vi "Query Multi Eval Meas Modulation Limit Check Results.vi"(8 "error in (no error)":errorcluster, 9 "Result Type (Current)":i32(ring) items=["Current", "Average", "Extreme"], 10 "Instance (1)":T1=1, 11 "VISA resource name":refnum<visa-resource-name>) -> (0 "error out":errorcluster, 1 "Modulation Limit Check Results":i32[](array[numeric]), 2 "Reliability":i32, 3 "VISA resource name out":refnum<visa-resource-name>)   [LabVIEW 2020, in "Rohde&Schwarz CMXP NR FR2 Measurement.lvlib"]
doc: "Starts a new single shot measurement and returns the multi eval measurement modulation results.\n\nAttributes:\nRSCMXPNRFR2M_ATTR_QUERY_MULTI_EVAL_MEASUREMENT_MODULATION_AVERAGE_LIMIT_CHECK_RESULTS\nRSCMXPNRFR2M_ATTR_QUERY_MULTI_EVAL_MEASUREMENT_MODULATION_CURRENT_LIMIT_CHECK_RESULTS\nRSCMXPNRFR2M_ATTR_QUERY_MULTI_EVAL_MEASUREMENT_MODULATION_EXTREME_LIMIT_CHECK_RESULTS\n\nRemote-control commands:\nCALCulate:NRMMw:MEAS<i>:MEValuation:MODulation:AVERage?\nCALCulate:NRMMw:MEAS<i>:MEValuation:MODulation:CURRent?\nCALCulate:NRMMw:MEAS<i>:MEValuation:MODulation:EXTReme?"
uses:
  <instrlib>/Rohde&Schwarz CMXP NR FR2 Measurement/Rohde&Schwarz CMXP NR FR2 Measurement.lvlib
  <instrlib>/Rohde&Schwarz CMXP NR FR2 Measurement/Private/_Instance.ctl
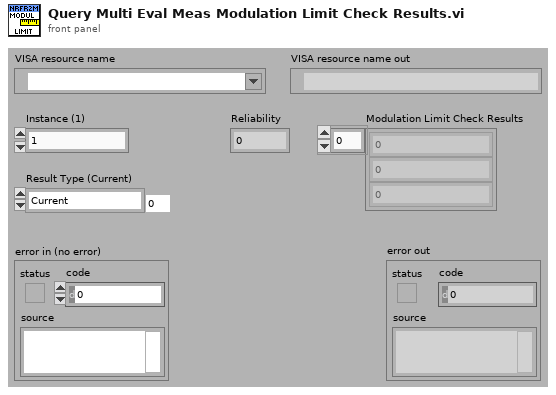
[diagram p1: front panel]
types:
  T1 = typedef "Rohde&Schwarz CMXP NR FR2 Measurement.lvlib/_Instance.ctl" = i32
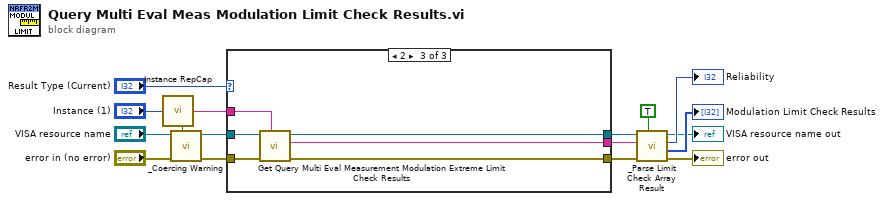
[diagram p0: block diagram]
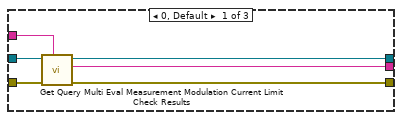
[diagram p2: hidden frame]
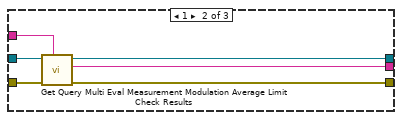
[diagram p3: hidden frame]
diagram:
  n1 = call <instrlib>:"Instance RepCap.vi"("Instance In"="Instance (1)") -> ("In Range?"=w5:bool, "RepCap Identifier Out"=w16:string)  [unwired: 1 in]
  n2 = call <instrlib>:"_Coercing Warning.vi"("In Range?"=w5, "error in (no error)"="error in (no error)", "VISA resource name"="VISA resource name") -> ("error out"=w3:errorcluster, "VISA resource name out"=w4:refnum<visa-resource-name>)  [unwired: 7 in]
  n3 = case shown="2" "Result Type (Current)" {
    tunnel: w16 -> [w22 w28 w34]
    tunnel: w3 -> [w21 w27 w33]
    tunnel: w4 -> [w20 w26 w32]
    tunnel: [w19 w25 w31] -> w15
    tunnel: [w18 w24 w30] -> w14
    tunnel: [w17 w23 w29] -> w13
    frame 0, Default {
      n4 = call "Get Query Multi Eval Measurement Modulation Current Limit Check Results"("Repeated Capabilities"=w22, "error in (no error)"=w21, "instrument handle"=w20) -> ("error out"=w19:errorcluster, "Query Multi Eval Measurement Modulation Current Limit Check Results"=w17:string, "instrument handle out"=w18:refnum<visa-resource-name>)  [unwired: 6 in]
    }
    frame 1 {
      n5 = call "Get Query Multi Eval Measurement Modulation Average Limit Check Results"("Repeated Capabilities"=w28, "error in (no error)"=w27, "instrument handle"=w26) -> ("error out"=w25:errorcluster, "Query Multi Eval Measurement Modulation Average Limit Check Results"=w23:string, "instrument handle out"=w24:refnum<visa-resource-name>)  [unwired: 6 in]
    }
    frame 2 {
      n6 = call "Get Query Multi Eval Measurement Modulation Extreme Limit Check Results"("Repeated Capabilities"=w34, "error in (no error)"=w33, "instrument handle"=w32) -> ("error out"=w31:errorcluster, "Query Multi Eval Measurement Modulation Extreme Limit Check Results"=w29:string, "instrument handle out"=w30:refnum<visa-resource-name>)  [unwired: 6 in]
    }
  }
  n7 = call <instrlib>:"_Parse Limit Check Array Result.vi"("error in (no error)"=w15, "Input String"=w13, "VISA resource name"=w14, "Out of tolerance? (F)"=TRUE ("Out of tolerance? (T)")) -> ("error out"=→"error out":errorcluster, "Results"=→"Modulation Limit Check Results":i32[], "Reliability"=→"Reliability":i32, "VISA resource name out"=→"VISA resource name out":refnum<visa-resource-name>)  [unwired: 3 in]
